vi "CVT Bool Read.vi"(3 "error in (no error)":errorcluster, 5 "Tag Name":string) -> (0 "error out":errorcluster, 1 "Value":bool)   [LabVIEW 2010]
uses:
  Current Value Table.lvlib
  DataTypes/Boolean_Read.vi
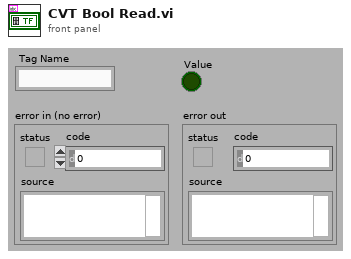
[diagram p1: front panel]
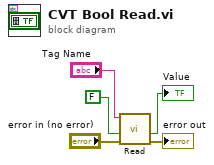
[diagram p0: block diagram]
diagram:
  n1 = call-poly "Read.vi"("error in (no error)"="error in (no error)", "Default"=FALSE, "Tag Name"="Tag Name") -> ("error out"=→"error out":errorcluster, "Value"=→"Value":bool)  [unwired: 7 in]
